vi "Data Server.vi"() -> ()   [LabVIEW 2011]
doc: "Sends a specified waveform through a TCP port. The VI first listens for a connection and, once established, sends the number of bytes to be sent followed by the data. After the data is sent, the VI waits for an 'all received' signal from the client and then breaks the connection.\n\n<B>Note:</B> Requires the Data Client.vi located in the same library as this VI."
panel:
  in  "stop":bool
  in  "Noise Level":dbl(slide)=0.36734693877551017 scale=0.0..1.0 scale format="%0.1f"
  in  "# of Points":i32=200
  in  "Function":u16(ring)=1 items=["random", "sine wave", "cosine wave"]
  in  "Port":u16=6340 min=1025 step=1
  # "Instructions:\n1. Open the Data Client.vi\n2. Run This VI first.\n3. Run the Data Client.vi Second.\n4. Adjust the # of Points Function, and Noise Level controls.\n5. Observe the Chart on the Data Client.vi.\n6. Stop This VI. The Data Client.vi will time out and stop."
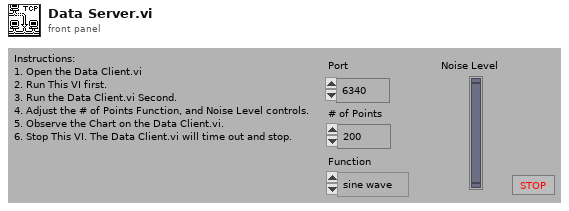
[diagram p1: front panel]
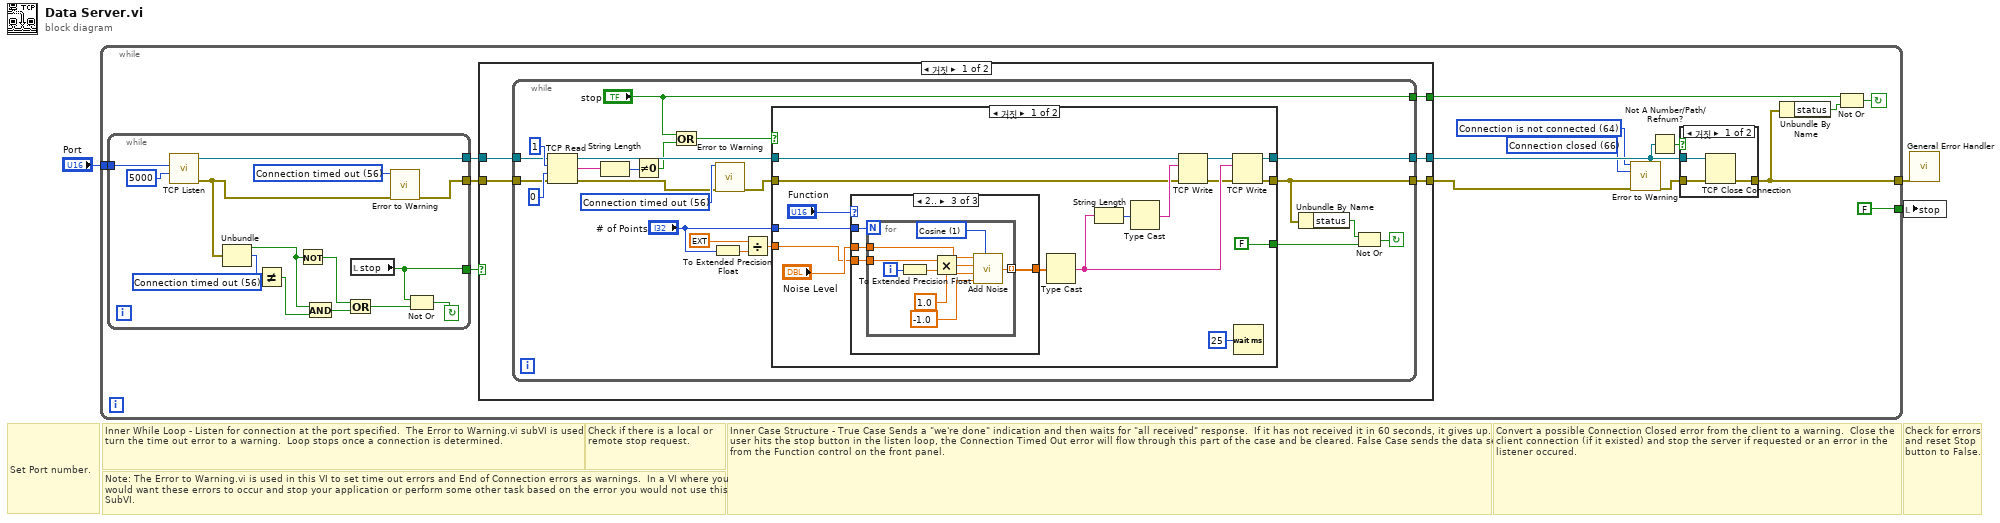
[diagram p0: block diagram]
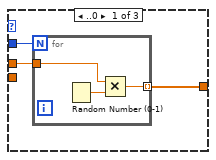
[diagram p2: hidden frame]
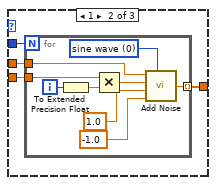
[diagram p3: hidden frame]
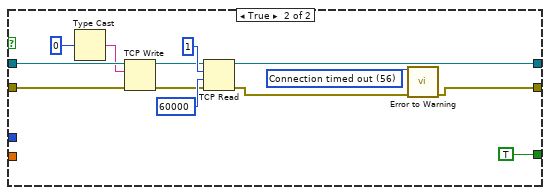
[diagram p4: hidden frame]
diagram:
  # "Check for errors\nand reset Stop \nbutton to False."
  # "Inner Case Structure - True Case Sends a \"we're done\" indication and then waits for \"all received\" response.  If it has not received it in 60 seconds, it gives up.  If the user hits the stop button in the listen loop, the Connection Timed Out error will flow through this part of the case and be cleared. False Case sends the data selected from the Function control on the front panel."
  # "Check if there is a local or remote stop request."
  # "Set Port number."
  # "Inner While Loop - Listen for connection at the port specified.  The Error to Warning.vi subVI is used to turn the time out error to a warning.  Loop stops once a connection is determined."
  # "Note: The Error to Warning.vi is used in this VI to set time out errors and End of Connection errors as warnings.  In a VI where you would want these errors to occur and stop your application or perform some other task based on the error you would not use this SubVI."
  # "Convert a possible Connection Closed error from the client to a warning.  Close the client connection (if it existed) and stop the server if requested or an error in the listener occured."
  n1 = while {
    tunnel: [w11] -> w2
    tunnel: "Port" -> [w17]
    tunnel: [FALSE] -> w1
    stop <- w18 continue-if-true
    w6 = 66 items=["No Error", "Argument Error", "Memory Full", "Out of Zone", "End of File", "File Already Open", "Generic File IO Error", "File Not Found", "File Permission Error", "Disk Full", "Duplicate Path", "Too Many Files Open", "Not Enabled", "Resource File Not Found", "Cannot Add Resource", "Resource Not Found", "Image Not Found", "Image Memory Error", "Pen Does Not Exist", "Config Bad Type", "Config Token Not Found", "Config Parse Error", "Config Memory Error", "Bad External Code Format", "Bad External Code Offset", "External Code Not Present", "Null Window", "Destroy Window Mixup", "Null Menu", "Print Aborted", "Bad Print Record", "Print Driver Error", "Windows Error During Print", "Memory Error During Print", "Print Dialog Error", "Generic Print Error", "Invalid Device Refnum", "Device Not Found", "Device Parameter Error", "Device Unit Error", "Can't Open Device", "Device Call Aborted", "Generic Error", "Cancelled By User", "Object ID Too Low", "Object ID Too High", "Object Not In Heap", "Unknown Heap", "Bad DefProc ID", "DefProc Not In Table", "Message Out Of Range", "Null Method", "Unknown Message", "Manager Call Not Supported", "Bad address", "Connection In progress", "Connection timed out", "Connection is already in progress", "Network attribute not supported", "Network error", "Address in use", "System out of memory", "Connection aborted", "Connection refused", "Connection is not connected", "Connection is already connected", "Connection closed", "Initialize error (interapplication manager)", "Bad occurrence", "Wait on unbound occurrence handler", "Occurrence queue overflow", "Bad path", "Semaphore not signaled", "Unrecognized type (interapplication manager)"] ("2nd Error to Convert")
    w7 = 64 items=["No Error", "Argument Error", "Memory Full", "Out of Zone", "End of File", "File Already Open", "Generic File IO Error", "File Not Found", "File Permission Error", "Disk Full", "Duplicate Path", "Too Many Files Open", "Not Enabled", "Resource File Not Found", "Cannot Add Resource", "Resource Not Found", "Image Not Found", "Image Memory Error", "Pen Does Not Exist", "Config Bad Type", "Config Token Not Found", "Config Parse Error", "Config Memory Error", "Bad External Code Format", "Bad External Code Offset", "External Code Not Present", "Null Window", "Destroy Window Mixup", "Null Menu", "Print Aborted", "Bad Print Record", "Print Driver Error", "Windows Error During Print", "Memory Error During Print", "Print Dialog Error", "Generic Print Error", "Invalid Device Refnum", "Device Not Found", "Device Parameter Error", "Device Unit Error", "Can't Open Device", "Device Call Aborted", "Generic Error", "Cancelled By User", "Object ID Too Low", "Object ID Too High", "Object Not In Heap", "Unknown Heap", "Bad DefProc ID", "DefProc Not In Table", "Message Out Of Range", "Null Method", "Unknown Message", "Manager Call Not Supported", "Bad address", "Connection In progress", "Connection timed out", "Connection is already in progress", "Network attribute not supported", "Network error", "Address in use", "System out of memory", "Connection aborted", "Connection refused", "Connection is not connected", "Connection is already connected", "Connection closed", "Initialize error (interapplication manager)", "Bad occurrence", "Wait on unbound occurrence handler", "Occurrence queue overflow", "Bad path", "Semaphore not signaled", "Unrecognized type (interapplication manager)"] ("1st Error to Convert")
    n2 = while {
      tunnel: [w19] -> w14
      tunnel: [w28] -> w15
      tunnel: [w32] -> w16
      tunnel: w17 -> [w33]
      stop <- w30 continue-if-true
      w26 = 56 items=["No Error", "Argument Error", "Memory Full", "Out of Zone", "End of File", "File Already Open", "Generic File IO Error", "File Not Found", "File Permission Error", "Disk Full", "Duplicate Path", "Too Many Files Open", "Not Enabled", "Resource File Not Found", "Cannot Add Resource", "Resource Not Found", "Image Not Found", "Image Memory Error", "Pen Does Not Exist", "Config Bad Type", "Config Token Not Found", "Config Parse Error", "Config Memory Error", "Bad External Code Format", "Bad External Code Offset", "External Code Not Present", "Null Window", "Destroy Window Mixup", "Null Menu", "Print Aborted", "Bad Print Record", "Print Driver Error", "Windows Error During Print", "Memory Error During Print", "Print Dialog Error", "Generic Print Error", "Invalid Device Refnum", "Device Not Found", "Device Parameter Error", "Device Unit Error", "Can't Open Device", "Device Call Aborted", "Generic Error", "Cancelled By User", "Object ID Too Low", "Object ID Too High", "Object Not In Heap", "Unknown Heap", "Bad DefProc ID", "DefProc Not In Table", "Message Out Of Range", "Null Method", "Unknown Message", "Manager Call Not Supported", "Bad address", "Connection In progress", "Connection timed out", "Connection is already in progress", "Network attribute not supported", "Network error", "Address in use", "System out of memory", "Connection aborted", "Connection refused", "Connection is not connected", "Connection is already connected", "Connection closed", "Initialize error (interapplication manager)", "Bad occurrence", "Wait on unbound occurrence handler", "Occurrence queue overflow", "Bad path", "Semaphore not signaled", "Unrecognized type (interapplication manager)"] ("1st Error to Convert")
      w27 = 56 items=["No Error", "Argument Error", "Memory Full", "Out of Zone", "End of File", "File Already Open", "Generic File IO Error", "File Not Found", "File Permission Error", "Disk Full", "Duplicate Path", "Too Many Files Open", "Not Enabled", "Resource File Not Found", "Cannot Add Resource", "Resource Not Found", "Image Not Found", "Image Memory Error", "Pen Does Not Exist", "Config Bad Type", "Config Token Not Found", "Config Parse Error", "Config Memory Error", "Bad External Code Format", "Bad External Code Offset", "External Code Not Present", "Null Window", "Destroy Window Mixup", "Null Menu", "Print Aborted", "Bad Print Record", "Print Driver Error", "Windows Error During Print", "Memory Error During Print", "Print Dialog Error", "Generic Print Error", "Invalid Device Refnum", "Device Not Found", "Device Parameter Error", "Device Unit Error", "Can't Open Device", "Device Call Aborted", "Generic Error", "Cancelled By User", "Object ID Too Low", "Object ID Too High", "Object Not In Heap", "Unknown Heap", "Bad DefProc ID", "DefProc Not In Table", "Message Out Of Range", "Null Method", "Unknown Message", "Manager Call Not Supported", "Bad address", "Connection In progress", "Connection timed out", "Connection is already in progress", "Network attribute not supported", "Network error", "Address in use", "System out of memory", "Connection aborted", "Connection refused", "Connection is not connected", "Connection is already connected", "Connection closed", "Initialize error (interapplication manager)", "Bad occurrence", "Wait on unbound occurrence handler", "Occurrence queue overflow", "Bad path", "Semaphore not signaled", "Unrecognized type (interapplication manager)"] ("1st Error to Convert")
      n3 = call <vilib>:"TCP Listen.vi"("timeout ms (wait forever: -1)"=5000, "port"=w33) -> ("error out"=w29:errorcluster, "connection ID"=w32:refnum<k5>)  [unwired: 5 in, 3 out]
      n4 = Unbundle(w29) -> ("status"=w24:bool, "code"=w25:i32)  [unwired: 1 out]
      n5 = Not Equal?(x=w25, y=w26) -> (x != y?=w23:bool)
      n6 = Not(x=w24) -> (.not. x?=w22:bool)
      n7 = And(x=w24, y=w23) -> (x .and. y?=w21:bool)
      n8 = Or(x=w22, y=w21) -> (x .or. y?=w20:bool)
      n9 = local read "stop"() -> (w19:bool)
      n10 = call <vilib>:"Error to Warning.vi"("1st Error to Convert"=w27, "error in"=w29) -> ("warning out"=w28:errorcluster)  [unwired: 13 in]
      n11 = Not Or(1:w20, 2:w19) -> (0:w30:bool)
    }
    n12 = case shown="거짓" w14 {
      selector: w14 -> [_ w122]
      tunnel: [w38 w123] -> w5
      tunnel: w16 -> [w37 w124]
      tunnel: w15 -> [w36 w123]
      tunnel: [w35 w124] -> w13
      tunnel: [w34 w122] -> w9
      frame False {
        n13 = while {
          tunnel: ["stop"] -> w34
          tunnel: w36 -> [w57]
          tunnel: [w47] -> w38
          tunnel: [w53] -> w35
          tunnel: w37 -> [w56]
          stop <- w60 continue-if-true
          w41 = 56 items=["No Error", "Argument Error", "Memory Full", "Out of Zone", "End of File", "File Already Open", "Generic File IO Error", "File Not Found", "File Permission Error", "Disk Full", "Duplicate Path", "Too Many Files Open", "Not Enabled", "Resource File Not Found", "Cannot Add Resource", "Resource Not Found", "Image Not Found", "Image Memory Error", "Pen Does Not Exist", "Config Bad Type", "Config Token Not Found", "Config Parse Error", "Config Memory Error", "Bad External Code Format", "Bad External Code Offset", "External Code Not Present", "Null Window", "Destroy Window Mixup", "Null Menu", "Print Aborted", "Bad Print Record", "Print Driver Error", "Windows Error During Print", "Memory Error During Print", "Print Dialog Error", "Generic Print Error", "Invalid Device Refnum", "Device Not Found", "Device Parameter Error", "Device Unit Error", "Can't Open Device", "Device Call Aborted", "Generic Error", "Cancelled By User", "Object ID Too Low", "Object ID Too High", "Object Not In Heap", "Unknown Heap", "Bad DefProc ID", "DefProc Not In Table", "Message Out Of Range", "Null Method", "Unknown Message", "Manager Call Not Supported", "Bad address", "Connection In progress", "Connection timed out", "Connection is already in progress", "Network attribute not supported", "Network error", "Address in use", "System out of memory", "Connection aborted", "Connection refused", "Connection is not connected", "Connection is already connected", "Connection closed", "Initialize error (interapplication manager)", "Bad occurrence", "Wait on unbound occurrence handler", "Occurrence queue overflow", "Bad path", "Semaphore not signaled", "Unrecognized type (interapplication manager)"] ("1st Error to Convert")
          n14 = TCP Read(connection ID=w56, bytes to read=1, error in (no error)=w57, 9:0) -> (connection ID out=w54:refnum<k5>, data out=w55:string, error out=w40:errorcluster)  [unwired: 1 in]
          n15 = String Length(string=w55) -> (length=w51:i32)
          n16 = Not Equal To 0?(x=w51) -> (x != 0?=w50:bool)
          n17 = Or(x="stop", y=w50) -> (x .or. y?=w49:bool)
          n18 = To Extended Precision Float(1:"# of Points") -> (0:w45:ext)
          n19 = call <vilib>:"Error to Warning.vi"("1st Error to Convert"=w41, "error in"=w40) -> ("warning out"=w39:errorcluster)  [unwired: 13 in]
          n20 = Divide(x=ext 6.283185307179586477, y=w45) -> (x/y=w42:ext)
          n21 = case shown="거짓" w49 {
            tunnel: w39 -> [w71 w117]
            tunnel: w54 -> [w70 w115]
            tunnel: [w69 w119] -> w53
            tunnel: [w68 w110] -> w47
            tunnel: [FALSE TRUE] -> w52
            tunnel: "# of Points" -> [w63 _]
            tunnel: w42 -> [w62 _]
            frame False {
              n22 = case shown="2.." "Function" {
                tunnel: w63 -> [w79 w86 w99]
                tunnel: [w78 w83 w96] -> w64
                tunnel: w62 -> [_ w85 w97]
                tunnel: "Noise Level" -> [w77 w84 w98]
                frame ..0 {
                  n23 = for {
                    N: w79 -> [_]
                    tunnel: [w80] -> w78 mode=indexing
                    tunnel: w77 -> [w82]
                    n24 = Random Number (0-1)() -> (number: 0 to 1=w81:dbl)
                    n25 = Multiply(x=w82, y=w81) -> (x*y=w80:dbl)
                  }
                }
                frame 1 {
                  n26 = for {
                    N: w86 -> [_]
                    tunnel: w85 -> [w94]
                    tunnel: w84 -> [w93]
                    tunnel: [w92] -> w83 mode=indexing
                    i -> [w95]
                    w87 = u16 0 items=["sine wave", "cosine wave"] ("Function")
                    n27 = To Extended Precision Float(1:w95) -> (0:w91:ext)
                    n28 = Multiply(x=w94, y=w91) -> (x*y=w88:ext)
                    n29 = call "Add Noise.vi"("noise"=w93, "input"=w88, "max"=1.0, "min"=-1.0, "Function"=w87) -> ("output"=w92:dbl)
                  }
                }
                frame 2.. {
                  n30 = for {
                    N: w99 -> [_]
                    tunnel: [w107] -> w96 mode=indexing
                    tunnel: w98 -> [w103]
                    tunnel: w97 -> [w102]
                    i -> [w108]
                    w100 = u16 1 items=["Sine", "Cosine"] ("Function")
                    n31 = To Extended Precision Float(1:w108) -> (0:w106:ext)
                    n32 = Multiply(x=w102, y=w106) -> (x*y=w101:ext)
                    n33 = call "Add Noise.vi"("noise"=w103, "input"=w101, "max"=1.0, "min"=-1.0, "Function"=w100) -> ("output"=w107:dbl)
                  }
                }
              }
              n34 = Type Cast(x=w64) -> (*(type *) &x=w76:string)  [unwired: 1 in]
              n35 = String Length(string=w76) -> (length=w74:i32)
              n36 = Type Cast(x=w74) -> (*(type *) &x=w75:string)  [unwired: 1 in]
              n37 = TCP Write(connection ID=w70, data in=w75, error in (no error)=w71) -> (connection ID out=w72:refnum<k5>, error out=w73:errorcluster)  [unwired: 1 in, 1 out]
              n38 = TCP Write(connection ID=w72, data in=w76, error in (no error)=w73) -> (connection ID out=w69:refnum<k5>, error out=w68:errorcluster)  [unwired: 1 in, 1 out]
              n39 = Wait (ms)(milliseconds to wait=u32 25) -> ()  [unwired: 1 out]
            }
            frame True {
              w109 = 56 items=["No Error", "Argument Error", "Memory Full", "Out of Zone", "End of File", "File Already Open", "Generic File IO Error", "File Not Found", "File Permission Error", "Disk Full", "Duplicate Path", "Too Many Files Open", "Not Enabled", "Resource File Not Found", "Cannot Add Resource", "Resource Not Found", "Image Not Found", "Image Memory Error", "Pen Does Not Exist", "Config Bad Type", "Config Token Not Found", "Config Parse Error", "Config Memory Error", "Bad External Code Format", "Bad External Code Offset", "External Code Not Present", "Null Window", "Destroy Window Mixup", "Null Menu", "Print Aborted", "Bad Print Record", "Print Driver Error", "Windows Error During Print", "Memory Error During Print", "Print Dialog Error", "Generic Print Error", "Invalid Device Refnum", "Device Not Found", "Device Parameter Error", "Device Unit Error", "Can't Open Device", "Device Call Aborted", "Generic Error", "Cancelled By User", "Object ID Too Low", "Object ID Too High", "Object Not In Heap", "Unknown Heap", "Bad DefProc ID", "DefProc Not In Table", "Message Out Of Range", "Null Method", "Unknown Message", "Manager Call Not Supported", "Bad address", "Connection In progress", "Connection timed out", "Connection is already in progress", "Network attribute not supported", "Network error", "Address in use", "System out of memory", "Connection aborted", "Connection refused", "Connection is not connected", "Connection is already connected", "Connection closed", "Initialize error (interapplication manager)", "Bad occurrence", "Wait on unbound occurrence handler", "Occurrence queue overflow", "Bad path", "Semaphore not signaled", "Unrecognized type (interapplication manager)"] ("1st Error to Convert")
              n40 = Type Cast(x=0) -> (*(type *) &x=w112:string)  [unwired: 1 in]
              n41 = TCP Write(connection ID=w115, data in=w112, error in (no error)=w117) -> (connection ID out=w114:refnum<k5>, error out=w116:errorcluster)  [unwired: 1 in, 1 out]
              n42 = TCP Read(connection ID=w114, bytes to read=1, error in (no error)=w116, 9:60000) -> (connection ID out=w119:refnum<k5>, error out=w111:errorcluster)  [unwired: 1 in, 1 out]
              n43 = call <vilib>:"Error to Warning.vi"("1st Error to Convert"=w109, "error in"=w111) -> ("warning out"=w110:errorcluster)  [unwired: 13 in]
            }
          }
          n44 = Unbundle By Name(w47) -> ("status"=w46:bool)
          n45 = Not Or(1:w52, 2:w46) -> (0:w60:bool)
        }
      }
      frame True {
      }
    }
    n46 = call <vilib>:"Error to Warning.vi"("1st Error to Convert"=w7, "2nd Error to Convert"=w6, "error in"=w5) -> ("warning out"=w4:errorcluster)  [unwired: 12 in]
    n47 = Not A Number/Path/Refnum?(number/path/refnum=w13) -> (NaN/Path/Refnum?=w12:bool)
    n48 = case shown="거짓" w12 {
      tunnel: w4 -> [w127 w128]
      tunnel: w13 -> [w126 _]
      tunnel: [w125 w128] -> w11
      frame False {
        n49 = TCP Close Connection(connection ID=w126, error in (no error)=w127) -> (error out=w125:errorcluster)  [unwired: 1 in, 1 out]
      }
      frame True {
      }
    }
    n50 = Unbundle By Name(w11) -> ("status"=w10:bool)
    n51 = Not Or(1:w10, 2:w9) -> (0:w18:bool)
  }
  n52 = local write "stop"(w1) -> ()
  n53 = call <vilib>:"General Error Handler.vi"("error in (no error)"=w2) -> ()  [unwired: 10 in, 5 out]
